vi "getReferenceDomainInfo.vi"(8 "error in (no error)":errorcluster, 11 "IDataDescriptor in":refnum<class "IDataDescriptor.lvclass">) -> (0 "error out":errorcluster, 2 "ReferenceDomainInfo out":refnum<class "IReferenceDomainInfo.lvclass">, 3 "IDataDescriptor out":refnum<class "IDataDescriptor.lvclass">)   [LabVIEW 2022 SP3, in "openDAQ.lvlib" / "IBaseObject.lvlib" / "IDataDescriptor.lvlib" / "IDataDescriptor.lvclass"]
uses:
  <instrlib>/openDAQ/Public/Classes/IDataDescriptor/IDataDescriptor.lvclass
  <instrlib>/openDAQ/Public/Classes/IDataDescriptor/IDataDescriptor.lvclass/IDataDescriptor.ctl
  <instrlib>/openDAQ/Public/Classes/IReferenceDomainInfo/IReferenceDomainInfo.lvclass
  <instrlib>/openDAQ/Binaries/Windows/x86/copendaq32.dll
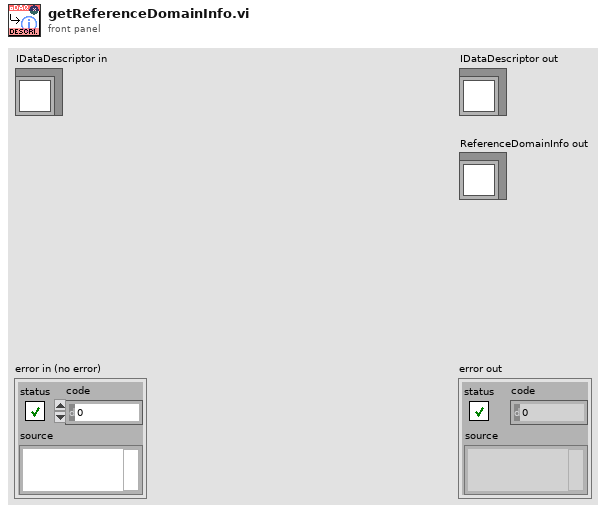
[diagram p1: front panel]
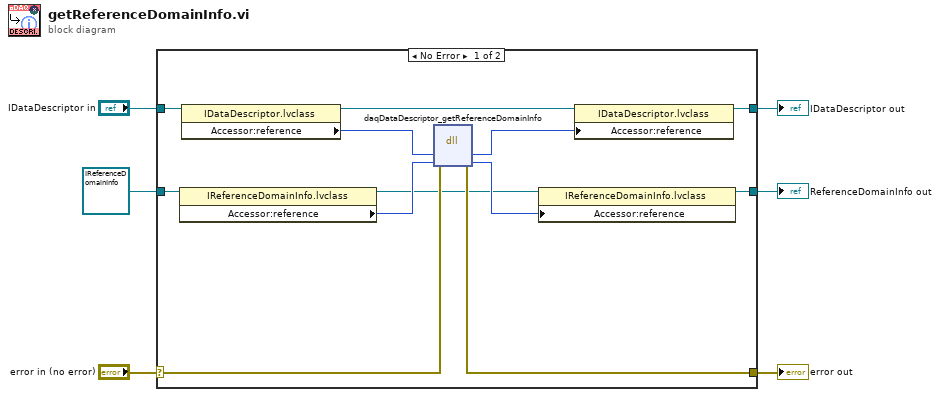
[diagram p0: block diagram]
diagram:
  n1 = case shown="No Error" "error in (no error)" {
    selector: "error in (no error)" -> [w16 w21]
    tunnel: [w15 w21] -> w5
    tunnel: [w10 w20] -> w3
    tunnel: "IDataDescriptor in" -> [w17 w20]
    tunnel: refnum<class "IReferenceDomainInfo.lvclass"> refnum ("openDAQ.lvlib:IBaseObject.lvlib:IReferenceDomainInfo.lvlib:IReferenceDomainInfo.lvclass") -> [w14 w19]
    tunnel: [w8 w19] -> w1
    frame No Error {
      n2 = property class="IReferenceDomainInfo.lvclass"(reference=w14) -> (reference out=w9:refnum<class "IReferenceDomainInfo.lvclass">, "Accessor:reference"=w12:i64)  [unwired: 1 in, 1 out]
      n3 = property class="IDataDescriptor.lvclass"(reference=w17) -> (reference out=w11:refnum<class "IDataDescriptor.lvclass">, "Accessor:reference"=w13:i64)  [unwired: 1 in, 1 out]
      n4 = dll-call lib="C:/Program Files (x86)/National Instruments/LabVIEW 2022/instr.lib/openDAQ/Binaries/Windows/x86/copendaq*.*" fn="daqDataDescriptor_getReferenceDomainInfo"(error in=w16, "dataDesriptior"=w13, "referenceDomainInfo"=w12) -> (error out=w15:errorcluster, "dataDesriptior"=w7:i64, "referenceDomainInfo"=w18:i64)  [unwired: 3 in, 1 out]
      n5 = property class="IReferenceDomainInfo.lvclass"(reference=w9, "Accessor:reference"=w18) -> (reference out=w8:refnum<class "IReferenceDomainInfo.lvclass">)  [unwired: 1 in, 1 out]
      n6 = property class="IDataDescriptor.lvclass"(reference=w11, "Accessor:reference"=w7) -> (reference out=w10:refnum<class "IDataDescriptor.lvclass">)  [unwired: 1 in, 1 out]
    }
    frame Error {
    }
  }
  "error out" <- w5
  "IDataDescriptor out" <- w3
  "ReferenceDomainInfo out" <- w1
